vi "Strommessung.vi"(5 "Spannung":dbl) -> (0 "Prozentualladung (unngenau)":dbl, 1 "Amperesekunde verbraucht":dbl=-149.04557758721205, 2 "Wattsekunde verbraucht":dbl=-149.04557758721205, 3 "Strom mit Abweichungen":dbl=-149.04557758721205)   [LabVIEW 2016]
uses:
  <vilib>/myRIO/Instrument Drivers/Onboard IO/AI/typedefs/AI Reference.ctl
  <vilib>/myRIO/Common/Instrument Driver Framework/Utilities/typedefs/myRIO Generic Hardware Reference.ctl
  <vilib>/myRIO/Common/Instrument Driver Framework/Utilities/typedefs/Hardware Version Enum.ctl
  <vilib>/myRIO/Common/Instrument Driver Framework/Utilities/typedefs/myRIO v1.0 Reference.ctl
  <vilib>/myRIO/Common/Instrument Driver Framework/Utilities/typedefs/Generic FPGA Reference.ctl
  <vilib>/myRIO/Common/Instrument Driver Framework/myRIO v1.0/AI/typedefs/AI Channels List.ctl
  <vilib>/myRIO/Common/Instrument Driver Framework/myRIO v1.0/AI/typedefs/AI Channels Enum.ctl
  <vilib>/myRIO/Common/Instrument Driver Framework/Utilities/typedefs/Analog Scaling Constants List.ctl
  <vilib>/myRIO/Common/Instrument Driver Framework/Utilities/typedefs/Analog Scaling Constants.ctl
  <vilib>/userdefined/High Color/nirio_resource_hc.ctl
  <vilib>/myRIO/Common/Instrument Driver Framework/Utilities/vis/Is FPGA Ref Available.vi
  <vilib>/myRIO/Common/Instrument Driver Framework/myRIO v1.0/AI/vis/myRIO v1.1 Open AI.vi
  <vilib>/myRIO/Instrument Drivers/Onboard IO/AI/vis/Read.vi
  <vilib>/myRIO/Common/Instrument Driver Framework/Utilities/vis/Validate Channels.vi
  <vilib>/myRIO/Common/Instrument Driver Framework/myRIO v1.0/AI/vis/myRIO v1.0 Reserve AI.vi
  <vilib>/myRIO/Common/Instrument Driver Framework/myRIO v1.0/AI/vis/myRIO v1.0 Build MUX Configuration AI.vi
  <vilib>/myRIO/Common/Instrument Driver Framework/myRIO v1.0/Resource Manager/vis/myRIO v1.0 Reserve Channel List.vi
  <vilib>/myRIO/Common/Instrument Driver Framework/myRIO v1.0/Resource Manager/vis/myRIO v1.0 Reserve Channel.vi
  <vilib>/myRIO/Common/Instrument Driver Framework/myRIO v1.0/Resource Manager/vis/myRIO v1.0 Unreserve Channel.vi
  <vilib>/myRIO/Common/Instrument Driver Framework/myRIO v1.0/Resource Manager/vis/myRIO v1.0 Build Mutex Name.vi
  <vilib>/Utility/VariantDataType/GetNumericInfo.vi
  <vilib>/Utility/error.llb/Error Cluster From Error Code.vi
  <vilib>/myRIO/Common/Instrument Driver Framework/myRIO v1.0/myRIO v1.1 Open.vi
  <vilib>/myRIO/Common/Instrument Driver Framework/myRIO v1.0/AI/vis/myRIO v1.0 Get Scaling Constants AI.vi
  <vilib>/myRIO/Common/Instrument Driver Framework/Utilities/vis/IO Manager.vi
  <vilib>/myRIO/Common/Instrument Driver Framework/Utilities/vis/Configuration Manager.vi
  <vilib>/myRIO/Common/Instrument Driver Framework/myRIO v1.0/myRIO v1.0 Close.vi
  <vilib>/myRIO/Common/Instrument Driver Framework/myRIO v1.0/AI/vis/myRIO v1.0 Read AI.vi
  <vilib>/myRIO/Express VI/Onboard IO/AI/AI Express VI.xnode
  <vilib>/myRIO/Instrument Drivers/Onboard IO/AI/vis/myRIO AI Open.xnode
  <vilib>/myRIO/Instrument Drivers/Onboard IO/AI/AI.lvlib
panel:
  out "Strom ohne Abweichung":dbl=-149.04557758721205
  out "Wahre Abweichung Mittelwert":dbl=-149.04557758721205
  out "Standartabweichung Strom\n+ -":dbl=-149.04557758721205
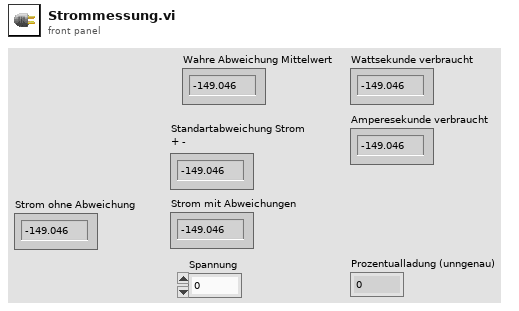
[diagram p1: front panel]
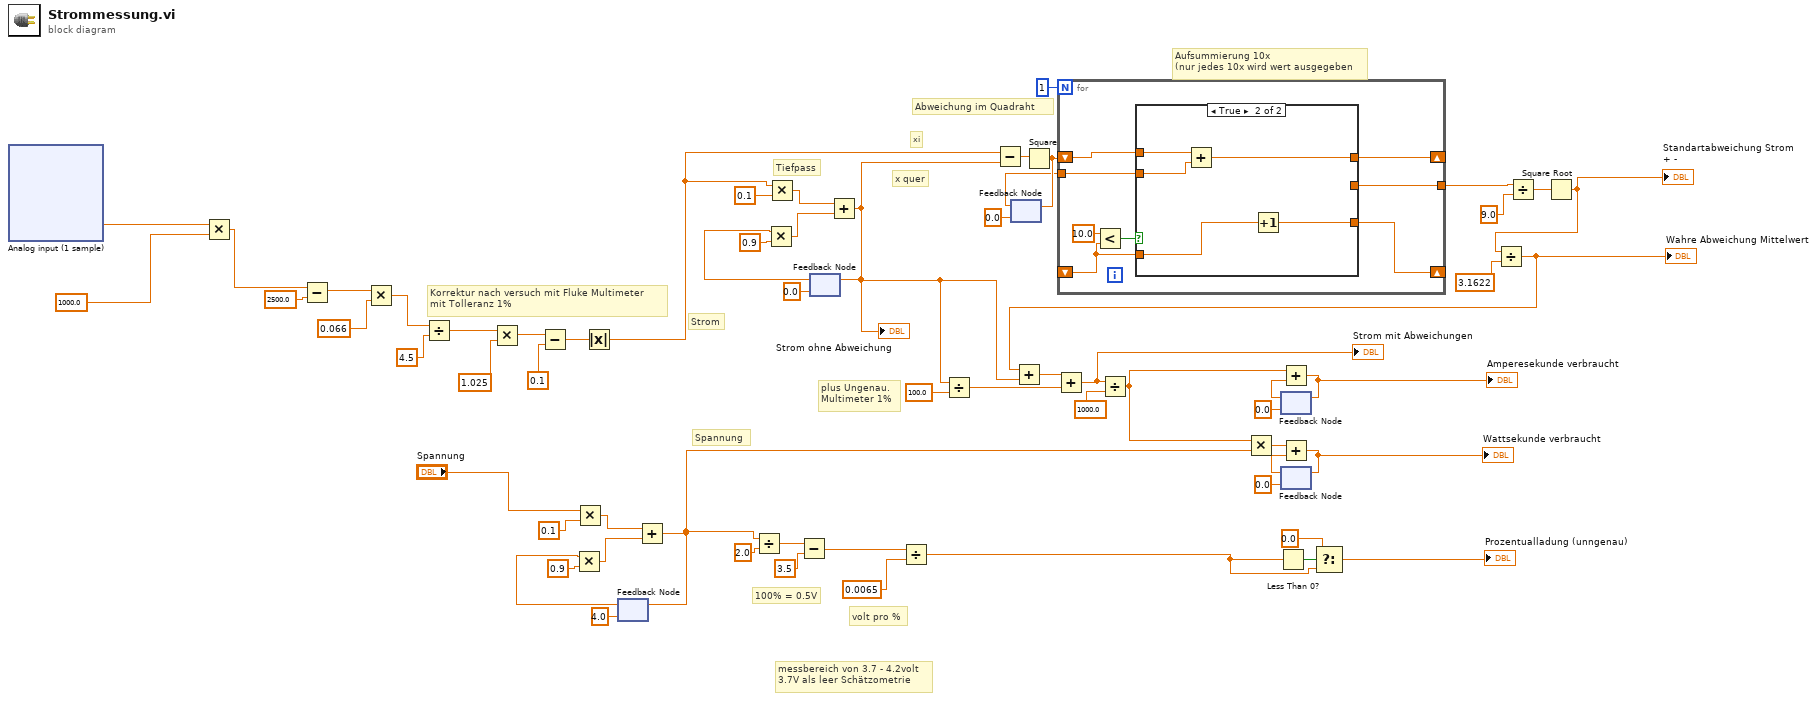
[diagram p0: block diagram]
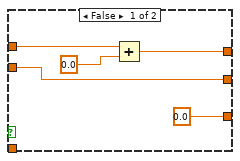
[diagram p2: hidden frame]
diagram:
  # "Spannung"
  # "Strom"
  # "Aufsummierung 10x\n(nur jedes 10x wird wert ausgegeben"
  # "plus Ungenau.\nMultimeter 1%"
  # "xi"
  # "x quer"
  # "Abweichung im Quadraht"
  # "Tiefpass"
  # "100% = 0.5V"
  # "messbereich von 3.7 - 4.2volt\n3.7V als leer Schätzometrie"
  # "volt pro %"
  # "Korrektur nach versuch mit Fluke Multimeter\nmit Tolleranz 1%"
  n1 = xnode "Analog input (1 sample)"() -> ("C/AI1 (AI1)"=w55:dbl)  [unwired: 1 in, 1 out]
  n2 = Multiply(x=w55, y=1000.0) -> (x*y=w60:dbl)
  n3 = Subtract(x=w60, y=2500.0) -> (x-y=w58:dbl)
  n4 = Multiply(x=w58, y=0.066) -> (x*y=w52:dbl)
  n5 = Divide(x=w52, y=4.5 ("x")) -> (x/y=w51:dbl)
  n6 = Multiply(x=w51, y=1.025) -> (x*y=w47:dbl)
  n7 = Subtract(x=w47, y=0.1) -> (x-y=w8:dbl)
  n8 = Multiply(x="Spannung", y=0.1) -> (x*y=w38:dbl)
  n9 = Absolute Value(x=w8) -> (abs(x)=w1:dbl)
  n10 = feedback #1(4.0) -> (w36:dbl)
  n11 = Multiply(x=w36, y=0.9) -> (x*y=w41:dbl)
  n12 = Add(x=w38, y=w41) -> (x+y=w26:dbl)
  n13 = feedback-in #1(w26) -> ()
  n14 = Divide(x=w26, y=2.0) -> (x/y=w31:dbl)
  n15 = Multiply(x=w1, y=0.1) -> (x*y=w48:dbl)
  n16 = Subtract(x=w31, y=3.5) -> (x-y=w29:dbl)
  n17 = feedback #2(0.0) -> (w54:dbl)
  n18 = Multiply(x=w54, y=0.9) -> (x*y=w62:dbl)
  n19 = Add(x=w48, y=w62) -> (x+y=w7:dbl)
  "Strom ohne Abweichung" <- w7
  n20 = feedback-in #2(w7) -> ()
  n21 = Divide(x=w29, y=0.0065) -> (x/y=w27:dbl)
  n22 = Divide(x=w7, y=100.0) -> (x/y=w9:dbl)
  n23 = Subtract(x=w1, y=w7) -> (x-y=w22:dbl)
  n24 = feedback #3(0.0) -> (w15:dbl)
  n25 = Square(x=w22) -> (x^2=w16:dbl)
  n26 = feedback-in #3(w16) -> ()
  n27 = for {
    N: 1 -> [_]
    shift-right: [w69] -> _
    shift-left: w16 -> [w70]
    shift-right: [w68] -> _
    shift-left: _ -> [w65]
    tunnel: w15 -> [w64]
    tunnel: [w63] -> w14
    n28 = Less?(x=10.0, y=w65) -> (x < y?=w66:bool)
    n29 = case shown="True" w66 {
      tunnel: w70 -> [w72 w80]
      tunnel: [w73 w77] -> w69
      tunnel: [0.0 w79] -> w68
      tunnel: w65 -> [_ w78]
      tunnel: w64 -> [w71 w76]
      tunnel: [w71 _] -> w63
      frame False {
        n30 = Add(x=w72, y=0.0) -> (x+y=w73:dbl)
      }
      frame True {
        n31 = Add(x=w80, y=w76) -> (x+y=w77:dbl)
        n32 = Increment(x=w78) -> (x+1=w79:dbl)
      }
    }
  }
  n33 = Less Than 0?(x=w27) -> (x < 0?=w34:bool)
  n34 = feedback #4(0.0) -> (w43:dbl)
  n35 = feedback #5(0.0) -> (w24:dbl)
  n36 = Select(t=0.0, s=w34, f=w27) -> (s? t:f=→"Prozentualladung (unngenau)":dbl)
  n37 = Divide(x=w14, y=9.0) -> (x/y=w13:dbl)
  n38 = Square Root(x=w13) -> (sqrt(x)=w18:dbl)
  "Standartabweichung Strom\n+ -" <- w18
  n39 = Divide(x=w18, y=3.1622) -> (x/y=w12:dbl)
  "Wahre Abweichung Mittelwert" <- w12
  n40 = Add(x=w12, y=w7) -> (x+y=w11:dbl)
  n41 = Add(x=w11, y=w9) -> (x+y=w6:dbl)
  "Strom mit Abweichungen" <- w6
  n42 = Divide(x=w6, y=1000.0) -> (x/y=w4:dbl)
  n43 = Multiply(x=w4, y=w26) -> (x*y=w23:dbl)
  n44 = Add(x=w4, y=w43) -> (x+y=w2:dbl)
  "Amperesekunde verbraucht" <- w2
  n45 = feedback-in #4(w2) -> ()
  n46 = Add(x=w23, y=w24) -> (x+y=w3:dbl)
  "Wattsekunde verbraucht" <- w3
  n47 = feedback-in #5(w3) -> ()
